vi "Example Threshold.vi"() -> ()   [LabVIEW 2013]
uses:
  C:/tf/play/labview/Tinkerforge.dll
  Tinkerforge.dll
panel:
  in  "stop":bool
  out "callback counter":i32
  out "last distance (cm)":i32
  in  "uid":string="amb"
  in  "port":i32=4223
  in  "host":string="localhost"
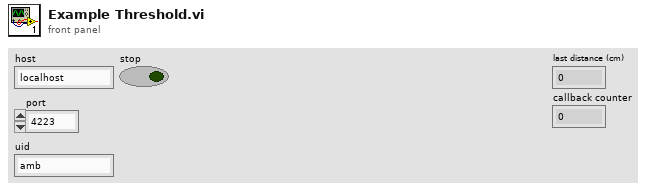
[diagram p1: front panel]
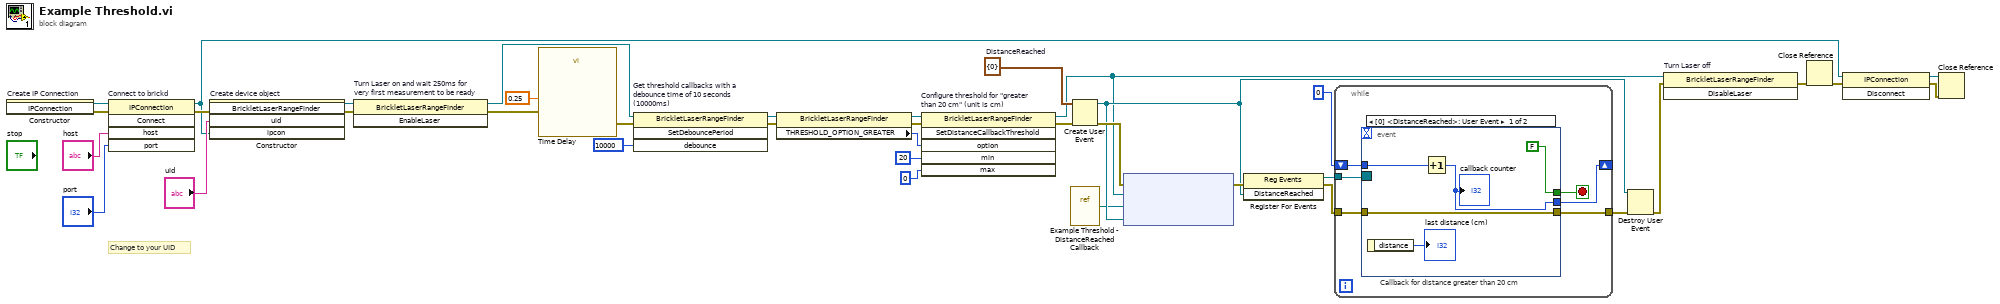
[diagram p0: block diagram]
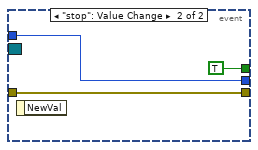
[diagram p2: hidden frame]
diagram:
  w22 = cluster{"distance":i32} {"distance"=0}  # DistanceReached
  # "Change to your UID"
  n1 = constructor on="Create IP Connection" class="IPConnection"() -> (reference out=w37:refnum<k24>, error out=w11:errorcluster)  [unwired: 3 in, 1 out]
  n2 = invoke on="Connect to brickd" class="IPConnection" method="Connect"(reference=w37, error in=w11, "host"="host", "port"="port") -> (reference out=w30:refnum<k24>, error out=w33:errorcluster)  [unwired: 1 in, 3 out]
  n3 = constructor on="Create device object" class="BrickletLaserRangeFinder"(error in=w33, "uid"="uid", "ipcon"=w30) -> (reference out=w8:refnum<k24>, error out=w10:errorcluster)  [unwired: 2 in, 3 out]
  n4 = invoke on="Turn Laser on and wait 250ms for\nvery first measurement to be ready" class="BrickletLaserRangeFinder" method="EnableLaser"(reference=w8, error in=w10) -> (reference out=w9:refnum<k24>, error out=w6:errorcluster)  [unwired: 1 in, 1 out]
  n5 = call "Time Delay"("error in (no error)"=w6, "Delay Time (s)"=0.25) -> ("error out"=w5:errorcluster)  [unwired: 9 in]
  n6 = invoke on="Get threshold callbacks with a\ndebounce time of 10 seconds\n(10000ms)" class="BrickletLaserRangeFinder" method="SetDebouncePeriod"(reference=w9, error in=w5, "debounce"=i64 10000 ("period")) -> (reference out=w15:refnum<k24>, error out=w17:errorcluster)  [unwired: 1 in, 2 out]
  n7 = property class="BrickletLaserRangeFinder"(reference=w15, error in=w17) -> (reference out=w14:refnum<k24>, error out=w16:errorcluster, "THRESHOLD_OPTION_GREATER"=w13:u16)
  n8 = invoke on="Configure threshold for \"greater\nthan 20 cm\" (unit is cm)" class="BrickletLaserRangeFinder" method="SetDistanceCallbackThreshold"(reference=w14, error in=w16, "option"=w13, "min"=20, "max"=0) -> (reference out=w2:refnum<k24>, error out=w20:errorcluster)  [unwired: 1 in, 4 out]
  n9 = vi-ref "Example Threshold - DistanceReached Callback.vi"() -> ("vi reference"=w1:refnum<vi>)
  n10 = Create User Event(user event datatype=w22, error in=w20) -> (user event=w23:refnum<user-event>, error out=w28:errorcluster)
  n11 = node ("Register Event Callback")(w28, w2, w1, w23) -> (w27:errorcluster)  [unwired: 1 in, 1 out]
  n12 = register-events(error in=w27, w23) -> (reference out=w26:refnum<event-registration>, error out=w24:errorcluster)  [unwired: 1 in]
  n13 = while {
    tunnel: w26 -> [w43]
    tunnel: [w42] -> w25
    tunnel: w24 -> [w41]
    shift-right: [w39] -> _
    shift-left: 0 -> [w40]
    stop <- w38 stop-if-true
    n14 = event "Callback for distance greater than 20 cm" shown="[0] <DistanceReached>: User Event" {
      selector: w43 -> [_ _]
      dyn-events: _ -> [_ _]
      timeout: _ -> [_ _]
      tunnel: [w48 w50] -> w42
      tunnel: w41 -> [w48 w50]
      tunnel: w40 -> [w47 w49]
      tunnel: [w46 w49] -> w39
      tunnel: [FALSE TRUE] -> w38
      event User Event {
        n15 = event-data() -> ("distance"=→"last distance (cm)":i32)  [unwired: 1 in]
        n16 = Increment(x=w47) -> (x+1=w46:i32)
        "callback counter" <- w46
      }
      event "stop": Value Change {
        n17 = event-data() -> ()  [unwired: 1 in, 1 out]
      }
    }
  }
  n18 = Destroy User Event(user event=w23, error in=w25) -> (error out=w4:errorcluster)
  n19 = invoke on="Turn Laser off" class="BrickletLaserRangeFinder" method="DisableLaser"(reference=w2, error in=w4) -> (error out=w3:errorcluster)  [unwired: 1 in, 2 out]
  n20 = Close Reference(error in (no error)=w3) -> (error out=w32:errorcluster)  [unwired: 1 in]
  n21 = invoke class="IPConnection" method="Disconnect"(reference=w30, error in=w32) -> (reference out=w29:refnum<k24>, error out=w31:errorcluster)  [unwired: 1 in, 1 out]
  n22 = Close Reference(reference=w29, error in (no error)=w31) -> ()  [unwired: 1 out]
